vi "Stop Core.vi"(10 "final error code":i32, 11 "DATABASE in":refnum<class "DATABASE.lvclass">) -> (3 "DATABASE out":refnum<class "DATABASE.lvclass">)   [LabVIEW 2019, in "DATABASE.lvlib" / "DATABASE.lvclass"]
doc: "(<B>Filename</B>: Actor Framework.lvlib:Actor.lvclass:Stop Core.vi)\n\nDefines what the actor does before it stops. Use the <B>final error code</B> input to determine whether the actor shut down in response to an error.\n\nBy default, this method passes the Stop message along to all auto-stop nested actors. A descendant class may override this method to define additional behavior, such as shutting down any processes the actor initiated in its override of the Actor Core method."
uses:
  DATABASE.lvclass
  <vilib>/ActorFramework/Actor/Actor.lvclass
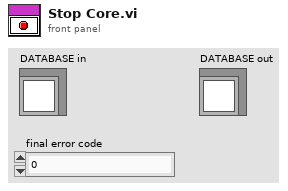
[diagram p1: front panel]
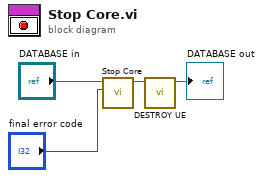
[diagram p0: block diagram]
diagram:
  n1 = call-parent "Stop Core.vi"("final error code"="final error code", "Actor in"="DATABASE in") -> ("Actor out"=w2:refnum<class "DATABASE.lvclass">)  [unwired: 9 in]
  n2 = call "DESTROY UE.vi"("DATABASE in"=w2) -> ("DATABASE out"=→"DATABASE out":refnum<class "DATABASE.lvclass">)  [unwired: 9 in, 1 out]
